vi "RT_AIChar.vi"() -> ()   [LabVIEW 2017]
uses:
  <vilib>/rvi/interface/nirviReadWriteControl/nirviReadWriteControl.xnode
  <vilib>/Platform/TimedLoop/XDataNode/XDataNode.xnode
  <vilib>/Platform/TimedLoop/XDataNode/nitl_modes.ctl
  <vilib>/Platform/TimedLoop/XDataNode/XDNodeRunTimeDep.lvlib
  <vilib>/Platform/TimedLoop/XDataNode/wakeup.ctl
  <vilib>/Platform/TimedLoop/XDataNode/timing_clust.ctl
  Components/Timing/Timing.lvlib
  <vilib>/rvi/interface/nirviOpenFPGA/nirviOpenFPGA.xnode
  <vilib>/NI/STM/NI STM.lvlib
  <vilib>/NI/STM/SubVIs/MetaDataElement.ctl
  <vilib>/NI/STM/TCP/Write Message (TCP).vi
  <vilib>/rvi/interface/Simulation/niFpgaSimulationCallBeginRW.vi
  <vilib>/rvi/errors/niLvFpgaAdjustHostInterfaceError.vi
  <vilib>/rvi/interface/nirviCloseFPGA/nirviCloseFPGA.xnode
  <vilib>/NI/STM/TCP/Write Meta Data (TCP Ref).vi
  <vilib>/NI/STM/TCP/Get Connection Reference (TCP).vi
  NiFpgaLv.dll
  <vilib>/Utility/error.llb/Error Cluster From Error Code.vi
  FPGA Bitfiles/flexlab_FPGATarget_Tbeam256MAMainVI_XFHOL9u-69o.lvbitx
  <vilib>/FPGAPlugInAG/Dynamic/niLvFpga_Close_Dynamic.vi
  <vilib>/FPGAPlugInAG/myRIO-1900/niLvFpga_Open_myRIO-1900.vi
  <vilib>/rvi/interface/common/dynamic/niFpgaDynamicAddResources.vi
panel:
  out "Sample Time\ntoo small?":bool
  in  "Run controller?":bool
  out "RT Loop Rate":dbl format="%.3p"
  out "# of iterations\n[STM write]":i32
  out "# elements \nFIFO buffer":u32
  out "Finished \nlate counter?":dbl
  in  "stop":bool
  # "- Open PC_SensorChar vi and run that VI as well to start capturing data!"
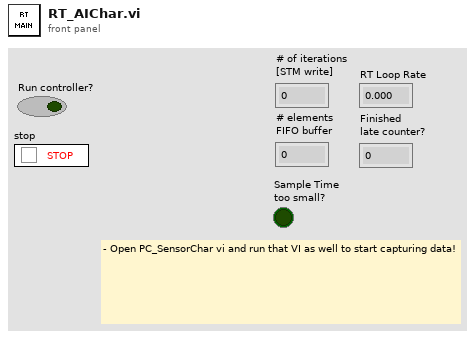
[diagram p1: front panel]
types:
  T1 = typedef "NI STM.lvlib/MetaDataElement.ctl" = string
  T2 = typedef "NI STM.lvlib/TCP Connection Info.ctl" = cluster{"connection ID":refnum<k5>, "meta data":T1[]}
  T3 = typedef "XDNodeRunTimeDep.lvlib/timing_clust.ctl" = cluster{"Expected End [f-1]":u64, "Actual End [f-1]":u64, "Finished Late? [f-1]":bool, "Expected End [i-1]":u64, "Actual End [i-1]":u64, "Finished Late? [i-1]":bool, "Expected Start [i]":u64, "Actual Start [i]":u64, "Expected Start [f]":u64, "Actual Start [f]":u64, "Source Name":string, "Structure Name":string, "Period":i64, "Deadline":i64, "Offset":i64, "Start":i64, "Priority":i32, "Timeout":i32, "Mode":T4, "Wakeup Reason":T5, "Error":errorcluster, "Source Type":string, "Secondary Source Type":string, "Global End Time":u64, "Global Start Time":u64, "Frame Duration":u64, "Iteration Duration":u64, "Assigned CPU":i32, "I/O Scan Engine Mode":u32}
  T4 = typedef "XDNodeRunTimeDep.lvlib/nitl_modes.ctl" = enum32{"No Change", "Process missed periods, maintain original phase", "Discard missed periods, maintain original phase", "Process missed periods, ignore original phase", "Discard missed periods, ignore original phase"}
  T5 = typedef "XDNodeRunTimeDep.lvlib/wakeup.ctl" = enum32{"Normal", "Aborted", "Asynchronous wakeup", "Timing source error", "Timed loop error", "Timeout"}
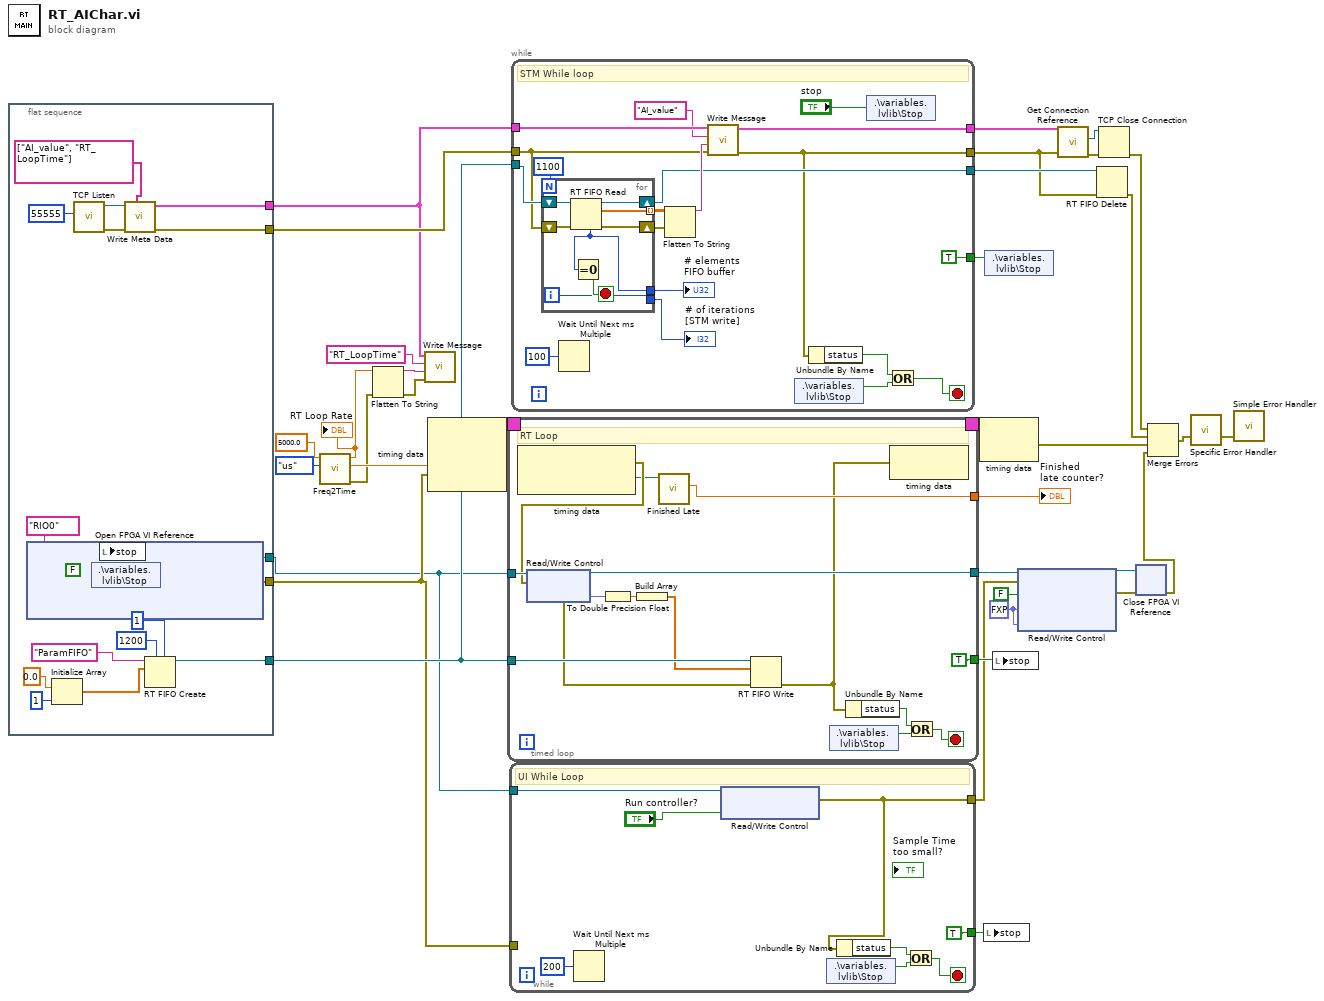
[diagram p0: block diagram]
diagram:
  w1 = fxp<+/-,26,4> 0.0 ("U_twist [V]")
  n1 = flat-sequence {
    tunnel: [w52] -> w9
    tunnel: [w51] -> w8
    tunnel: [w46] -> w22
    tunnel: [w45] -> w30
    tunnel: [w44] -> w26
    frame #0 {
      w53 = FALSE ("Stop")
      n2 = xnode "Open FPGA VI Reference"("resource name"=tag "RIO0") -> ("FPGA VI Reference Out"=w51:refnum<k20>, "error out"=w54:errorcluster)  [unwired: 1 in]
      n3 = Initialize Array(0.0 ("element"), 1 ("dimension size")) -> (w39:dbl[])
      n4 = call <vilib>:"TCP Listen.vi"("port"=u16 55555) -> ("error out"=w49:errorcluster, "connection ID"=w48:refnum<k5>)  [unwired: 6 in, 3 out]
      n5 = shared-variable ".\\variables.lvlib\\Stop"(w53, error in=w54) -> (error out=w52:errorcluster)
      n6 = local write "stop"(w53) -> ()
      n7 = call-poly <vilib>:"Write Meta Data.vi"("meta data"=T1[] ["AI_value", "RT_LoopTime"], "error in"=w49, "connection ID"=w48) -> ("error out"=w45:errorcluster, "connection info out"=w46:T2)  [unwired: 7 in]
      n8 = RT FIFO Create(0:"ParamFIFO" ("name (unnamed)"), 1:w39, 4:u32 1200 ("size (10)"), 6:u32 1 ("elements in array (1)")) -> (8:w44:refnum<k33>)  [unwired: 4 in, 2 out]
    }
  }
  n9 = call "Freq2Time.vi"("Int. Time Unit"=enum16{"sec", "us", "ms"}."us", "Sample rate (Hz)"=5000.0 ("Period")) -> ("error out"=w16:errorcluster, "Int.  time [unit]"=w31:dbl, "New Sample rate (Hz)"=w18:dbl)  [unwired: 7 in]
  "RT Loop Rate" <- w18
  n10 = Flatten To String(anything=w18, error in (no error)=w16) -> (data string=w19:string, error out=w20:errorcluster)  [unwired: 2 in, 1 out]
  n11 = call-poly <vilib>:"Write Message.vi"("error in"=w20, "data"=w19, "name"="RT_LoopTime", "connection info in"=w22) -> ()  [unwired: 6 in, 2 out]
  n12 = node-c288(w31, w9) -> (w36:T3)  [unwired: 1 in]
  n13 = timed-loop {
    tunnel: w8 -> [w69]
    timing: w36 -> [_]
    timing-out: [_] -> w35
    tunnel: [w66] -> w34
    tunnel: w26 -> [w65]
    tunnel: [TRUE ("Stop")] -> w6
    tunnel: [w59] -> w7
    stop <- w58 stop-if-true
    # "RT Loop"
    n14 = node-c288() -> (w68:errorcluster, w67:bool)  [unwired: 1 in]
    n15 = xnode "Read/Write Control"("FPGA VI Reference In"=w69, "error in"=w68) -> ("FPGA VI Reference Out"=w59:refnum<k20>, "error out"=w60:errorcluster, "Hall2 [V]"=w64:fxp<+,25,3>)
    n16 = To Double Precision Float(number=w64) -> (double precision float=w63:dbl)
    n17 = Build Array(w63) -> (w62:dbl[])
    n18 = call "Finished Late.vi"("Finished \nLate?"=w67) -> ("# Finished\nLate counter"=w66:dbl)  [unwired: 8 in, 2 out]
    n19 = RT FIFO Write(0:w65, 1:w62, 3:w60) -> (11:w55:errorcluster)  [unwired: 2 in, 3 out]
    n20 = shared-variable ".\\variables.lvlib\\Stop"() -> (w57:bool)  [unwired: 1 in, 1 out]
    n21 = Unbundle By Name(w55) -> ("status"=w56:bool)
    n22 = node-c288(w55) -> ()  [unwired: 1 out]
    n23 = Or(x=w56, y=w57) -> (x .or. y?=w58:bool)
  }
  "Finished \nlate counter?" <- w34
  n24 = while {
    tunnel: w9 -> [_]
    tunnel: w8 -> [w81]
    tunnel: [TRUE ("Stop")] -> w5
    tunnel: [w76] -> w4
    stop <- w78 stop-if-true
    # "UI While Loop"
    n25 = Wait Until Next ms Multiple(millisecond multiple=u32 200) -> ()  [unwired: 1 out]
    n26 = xnode "Read/Write Control"("FPGA VI Reference In"=w81, "Run controller?"="Run controller?") -> ("error out"=w76:errorcluster)  [unwired: 1 in, 1 out]
    n27 = shared-variable ".\\variables.lvlib\\Stop"() -> (w79:bool)  [unwired: 1 in, 1 out]
    n28 = Unbundle By Name(w76) -> ("status"=w77:bool)
    n29 = Or(x=w77, y=w79) -> (x .or. y?=w78:bool)
  }
  n30 = while {
    tunnel: w22 -> [w101]
    tunnel: w30 -> [w94]
    tunnel: [w99] -> w29
    tunnel: [w84] -> w24
    tunnel: w26 -> [w96]
    tunnel: [w93] -> w25
    tunnel: [TRUE ("Stop")] -> w2
    stop <- w86 stop-if-true
    # "STM While loop"
    n31 = for {
      N: 1100 -> [_]
      shift-right: [w107] -> w93
      shift-left: w96 -> [w110]
      shift-right: [w109] -> w95
      shift-left: w94 -> [w108]
      tunnel: [w106] -> w92
      tunnel: [w104] -> w91
      tunnel: [w103] -> w90 mode=indexing
      i -> [w104]
      stop <- w105 stop-if-true
      n32 = RT FIFO Read(0:w110, 3:w108) -> (7:w106:u32, 8:w107:refnum<k33>, 9:w103:dbl[], 11:w109:errorcluster)  [unwired: 2 in, 1 out]
      n33 = Equal To 0?(x=w106) -> (x = 0?=w105:bool)
    }
    "# elements \nFIFO buffer" <- w92
    "# of iterations\n[STM write]" <- w91
    n34 = Wait Until Next ms Multiple(millisecond multiple=u32 100) -> ()  [unwired: 1 out]
    n35 = Flatten To String(anything=w90, error in (no error)=w95) -> (data string=w98:string)  [unwired: 2 in, 2 out]
    n36 = call-poly <vilib>:"Write Message.vi"("error in"=w94, "data"=w98, "name"="AI_value", "connection info in"=w101) -> ("error out"=w84:errorcluster, "connection info out"=w99:T2)  [unwired: 6 in]
    n37 = shared-variable ".\\variables.lvlib\\Stop"() -> (w87:bool)  [unwired: 1 in, 1 out]
    n38 = Unbundle By Name(w84) -> ("status"=w85:bool)
    n39 = shared-variable ".\\variables.lvlib\\Stop"("stop") -> ()  [unwired: 1 in, 1 out]
    n40 = Or(x=w85, y=w87) -> (x .or. y?=w86:bool)
  }
  n41 = node-c288(w35) -> (w17:errorcluster)
  n42 = local write "stop"(w5) -> ()
  n43 = shared-variable ".\\variables.lvlib\\Stop"(w2) -> ()  [unwired: 1 in, 1 out]
  n44 = local write "stop"(w6) -> ()
  n45 = xnode "Read/Write Control"("FPGA VI Reference In"=w7, "error in"=w4, "Run controller?"=FALSE ("AO enabled?"), "U_twist [V]"=w1, "U_bend [V]"=w1) -> ("FPGA VI Reference Out"=w12:refnum<k20>, "error out"=w11:errorcluster)
  n46 = call-poly <vilib>:"Get Connection Reference.vi"("error in"=w24, "connection info in"=w29) -> ("error out"=w28:errorcluster, "connection ID out"=w27:refnum<k5>)  [unwired: 7 in, 1 out]
  n47 = RT FIFO Delete(0:w25, 3:w24) -> (11:w23:errorcluster)  [unwired: 1 in]
  n48 = TCP Close Connection(connection ID=w27, error in (no error)=w28) -> (error out=w13:errorcluster)  [unwired: 1 in, 1 out]
  n49 = xnode "Close FPGA VI Reference"("FPGA VI Reference In"=w12, "error in"=w11) -> ("error out"=w3:errorcluster)
  n50 = Merge Errors(w13, w23, w17, w3) -> (w15:errorcluster)
  n51 = call "Specific Error Handler"("Error to Check"=w15) -> ("error out"=w14:errorcluster)  [unwired: 11 in, 3 out]
  n52 = call <vilib>:"Simple Error Handler.vi"("error in (no error)"=w14) -> ()  [unwired: 4 in, 5 out]
